vi "DAQ Performance Test.vi"() -> ()   [LabVIEW 2021]
uses:
  <vilib>/Platform/TimedLoop/XDataNode/wakeup.ctl
  <vilib>/Platform/TimedLoop/XDataNode/XDNodeRunTimeDep.lvlib
  <vilib>/Platform/TimedLoop/XDataNode/nitl_modes.ctl
  <vilib>/Platform/TimedLoop/XDataNode/timing_clust.ctl
  <vilib>/Platform/TimedLoop/XDataNode/XDataNode.xnode
  CIFChannels/Typedef/Direction.ctl
  CIFChannels/CIFChannels.lvclass
  ChannelCommon/typedef/FIFO Config.ctl
  ChannelCommon/ChannelCommon.lvlib
  CIF_CIPC_Fifo_DAQ.lvclass
  D:/dev/Packages/CIF_Channels_Core/src/CIPC_Channels/CIF_CIPC_Chan/CIF_CIPC_Chn.lvclass
  D:/dev/Packages/CIF_Channels_Core/src/CIFChannels/CIFChannels.lvclass
  D:/dev/Packages/CIF_Channels_Core/src/CIPC_Channels/FIFO_DAQ/CIF_CIPC_Fifo_DAQ.lvclass
  ChannelCommon/typedef/TimeStamps.ctl
  ChannelCommon/typedef/Datatype Waveform.ctl
  ChannelCommon/typedef/New FIFO Instance Configuration.ctl
  ChannelCommon/typedef/Benchmark Stats.ctl
panel:
  in  "stop":bool
  out "Flatten (us) TO":T1
  out "Channel R/W (us) TO":T1
  out "Flatten (us)":T1
  out "Channel R/W (us)":T1
  out "avg TO":dbl
  out "max TO":dbl
  out "timed out? 3":bool
  out "timed out?":bool
  out "avg channel":dbl
  out "max channel":dbl
  out "pass":bool
  out "error out":errorcluster
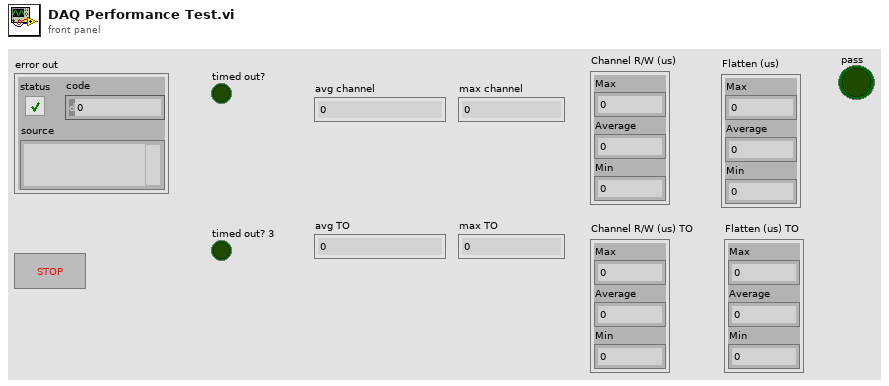
[diagram p1: front panel]
types:
  T1 = typedef "ChannelCommon.lvlib/Benchmark Stats.ctl" = cluster{"Max":i64, "Average":dbl, "Min":i64}
  T2 = typedef "ChannelCommon.lvlib/FIFO Config.ctl" = cluster{"Max Bytes/Msg":u64, "Max Msg/FIFO":u64, "Flags":u64}
  T3 = typedef "CIFChannels.lvclass/Direction.ctl" = enum16{"Publisher", "Subscriber"}
  T4 = typedef "ChannelCommon.lvlib/New FIFO Instance Configuration.ctl" = cluster{"Backpressure":bool, "Bytes/Message Override":u32, "Messages/FIFO Override":u32, "Custom Data":u8[]}
  T5 = typedef "ChannelCommon.lvlib/Datatype Waveform.ctl" = cluster{"Measurement":dbl[], "dT":dbl, "Timestamp":i64}
  T6 = typedef "ChannelCommon.lvlib/TimeStamps.ctl" = cluster{"ClockID":u8, "T0":i64, "T_Out":i64}
  T7 = typedef "XDNodeRunTimeDep.lvlib/timing_clust.ctl" = cluster{"Expected End [f-1]":u64, "Actual End [f-1]":u64, "Finished Late? [f-1]":bool, "Expected End [i-1]":u64, "Actual End [i-1]":u64, "Finished Late? [i-1]":bool, "Expected Start [i]":u64, "Actual Start [i]":u64, "Expected Start [f]":u64, "Actual Start [f]":u64, "Source Name":string, "Structure Name":string, "Period":i64, "Deadline":i64, "Offset":i64, "Start":i64, "Priority":i32, "Timeout":i32, "Mode":T8, "Wakeup Reason":T9, "Error":errorcluster, "Source Type":string, "Secondary Source Type":string, "Global End Time":u64, "Global Start Time":u64, "Frame Duration":u64, "Iteration Duration":u64, "Assigned CPU":i32, "I/O Scan Engine Mode":u32}
  T8 = typedef "XDNodeRunTimeDep.lvlib/nitl_modes.ctl" = enum32{"No Change", "Process missed periods, maintain original phase", "Discard missed periods, maintain original phase", "Process missed periods, ignore original phase", "Discard missed periods, ignore original phase"}
  T9 = typedef "XDNodeRunTimeDep.lvlib/wakeup.ctl" = enum32{"Normal", "Aborted", "Asynchronous wakeup", "Timing source error", "Timed loop error", "Timeout"}
  T10 = typedef "ChannelCommon.lvlib/New FIFO Instance Response.ctl" = cluster{"Publisher":string, "Custom Data":u8[]}
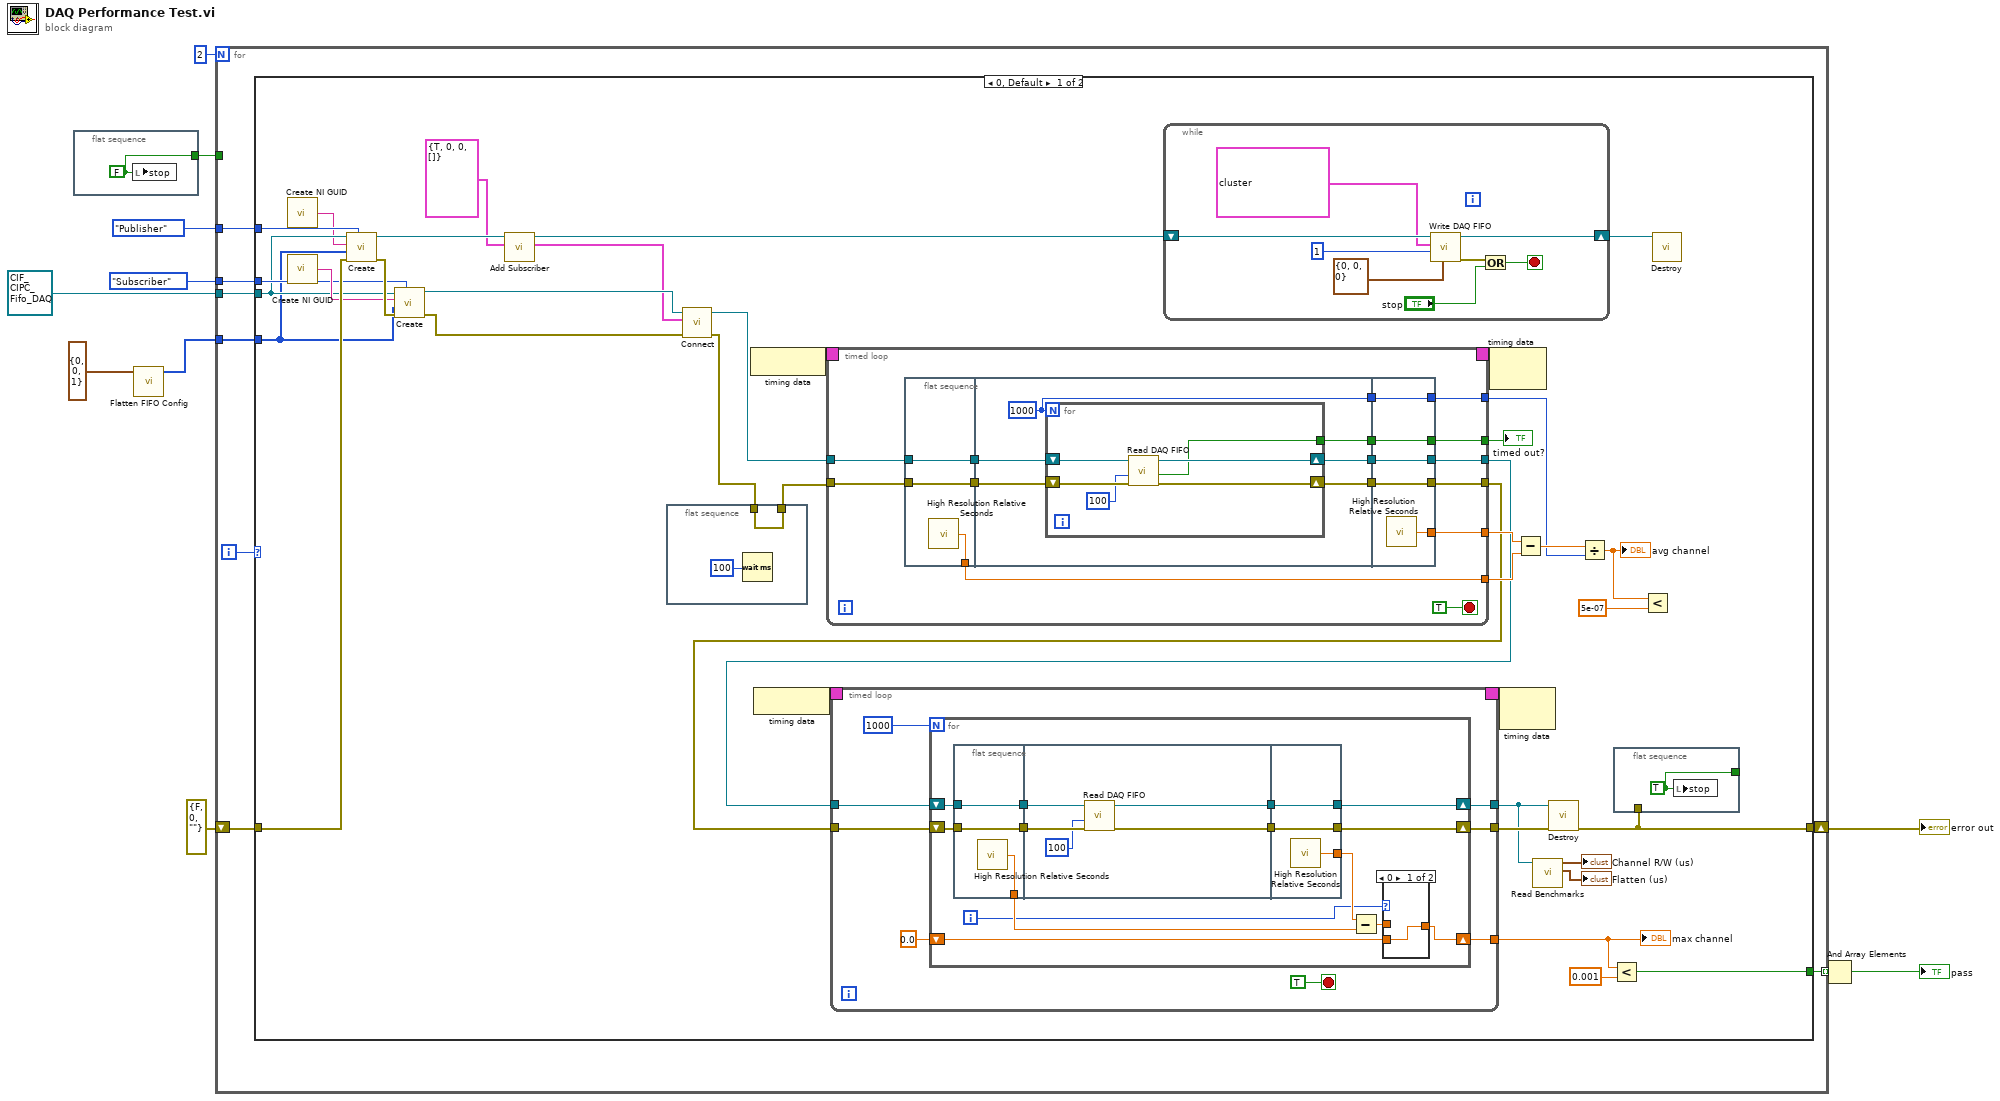
[diagram p0: block diagram]
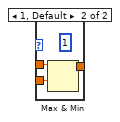
[diagram p2: hidden frame]
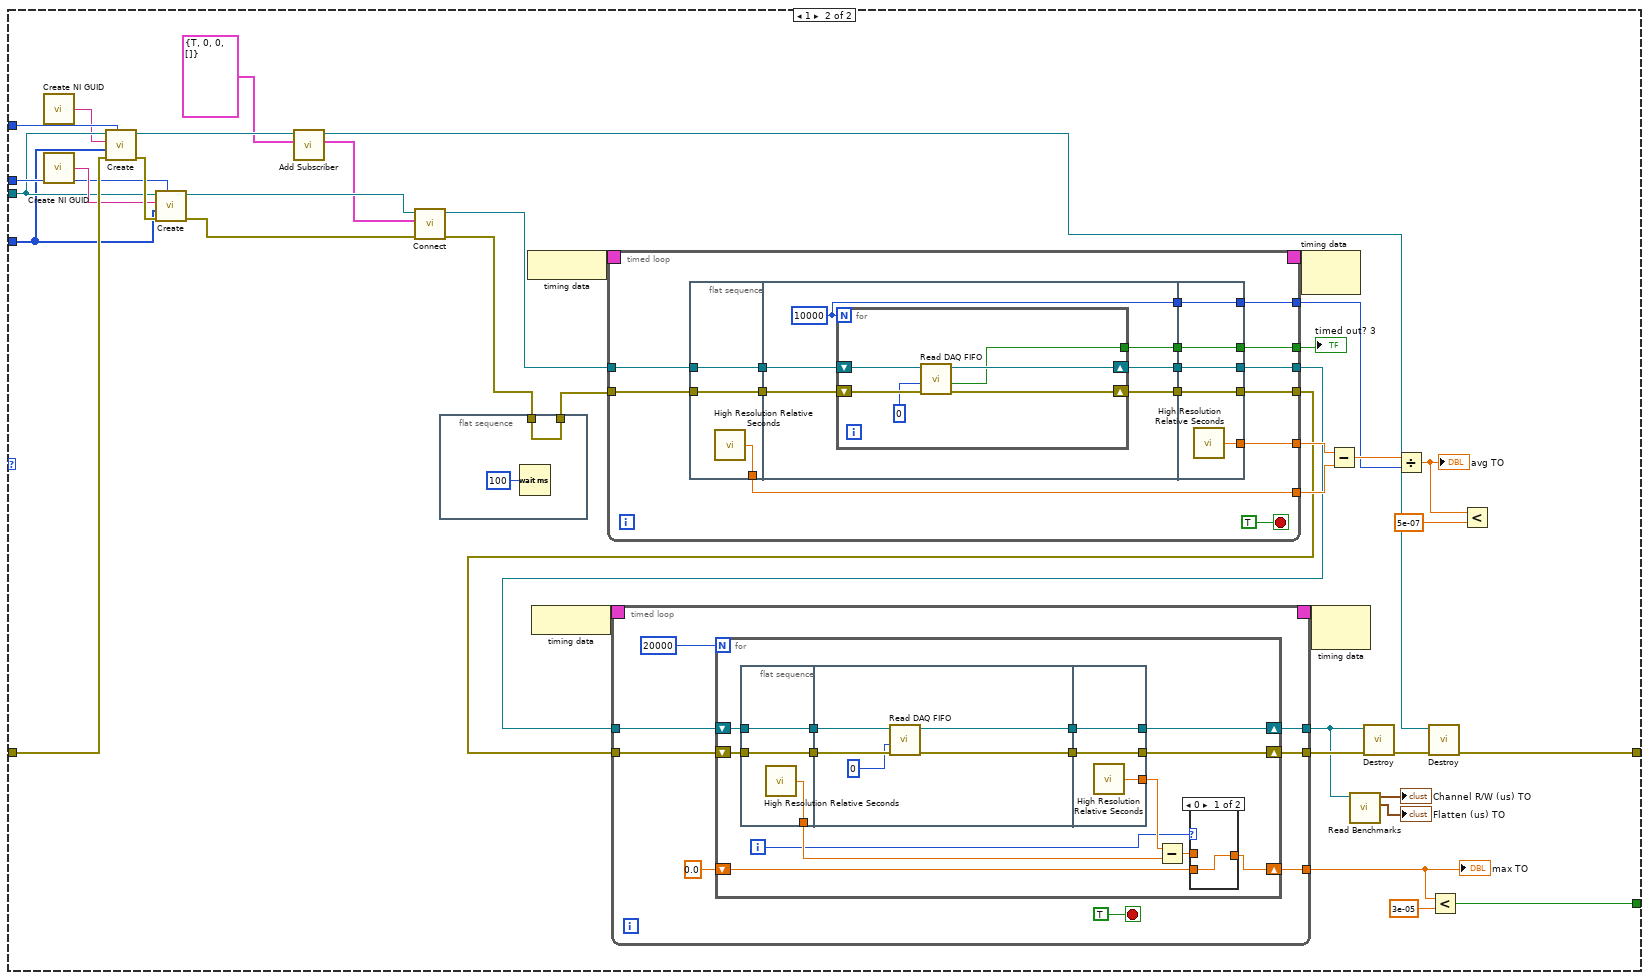
[diagram p3: hidden frame]
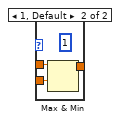
[diagram p4: hidden frame]
diagram:
  n1 = flat-sequence {
    tunnel: [w12] -> w1
    frame #0 {
      w12 = FALSE ("stop")
      n2 = local write "stop"(w12) -> ()
    }
  }
  n3 = call "Flatten FIFO Config.vi"("FIFO Config in"=T2 {"Max Bytes/Msg"=0, "Max Msg/FIFO"=0, "Flags"=1}) -> ("Flattened FIFO Config"=w3:u8[])  [unwired: 10 in]
  n4 = for {
    N: 2 -> [_]
    tunnel: [w20] -> w9 mode=indexing
    shift-right: [w19] -> w11
    shift-left: errorcluster {"status"=FALSE, "code"=0, "source"=""} ("error out") -> [w17]
    tunnel: Direction."Publisher" ("Direction") -> [w16]
    tunnel: Direction."Subscriber" ("Direction") -> [w15]
    tunnel: refnum<class "CIF_CIPC_Fifo_DAQ.lvclass"> refnum ("CIF_CIPC_Fifo_U8.lvclass") -> [w14]
    tunnel: w3 -> [w13]
    tunnel: w1 -> [_]
    i -> [w18]
    n5 = case shown="0, Default" w18 {
      tunnel: [w45 w175] -> w20
      tunnel: [w26 w161] -> w19
      tunnel: w17 -> [w43 w173]
      tunnel: w16 -> [w41 w171]
      tunnel: w15 -> [w40 w170]
      tunnel: w14 -> [w39 w169]
      tunnel: w13 -> [w36 w165]
      frame 0, Default {
        n6 = call <vilib>:"Create NI GUID.vi"() -> ("NI GUID"=w23:string)
        n7 = call <vilib>:"Create NI GUID.vi"() -> ("NI GUID"=w42:string)
        n8 = call-dynamic "Create.vi"("Direction"=w41, "error in (no error)"=w43, "Custom Config Data"=w36, "Name"=w23, "CIFFIFO in"=w39) -> ("error out"=w44:errorcluster, "CIFFIFO out"=w25:refnum<class "CIF_CIPC_Fifo_DAQ.lvclass">)  [unwired: 5 in]
        n9 = call-dynamic "Create.vi"("Direction"=w40, "error in (no error)"=w44, "Custom Config Data"=w36, "Name"=w42, "CIFFIFO in"=w39) -> ("error out"=w37:errorcluster, "CIFFIFO out"=w38:refnum<class "CIF_CIPC_Fifo_DAQ.lvclass">)  [unwired: 5 in]
        n10 = call-dynamic "Add Subscriber.vi"("New FIFO Instance Config"=T4 {"Backpressure"=TRUE, "Bytes/Message Override"=0, "Messages/FIFO Override"=0, "Custom Data"=[]}, "CIF_CIPC_Chn in"=w25) -> ("New FIFO Instance"=w22:T10, "CIF_CIPC_Chn out"=w24:refnum<class "CIF_CIPC_Fifo_DAQ.lvclass">)  [unwired: 7 in, 1 out]
        n11 = flat-sequence {
          tunnel: w33 -> [w62]
          tunnel: [w62] -> w32
          frame #0 {
            n12 = Wait (ms)(milliseconds to wait=u32 100) -> ()  [unwired: 1 out]
          }
        }
        n13 = call-dynamic "Connect.vi"("error in (no error)"=w37, "Connection"=w22, "CIFTag in"=w38) -> ("error out"=w33:errorcluster, "CIFTag out"=w35:refnum<class "CIF_CIPC_Fifo_DAQ.lvclass">)  [unwired: 7 in]
        n14 = node-c288() -> (w59:T7)
        n15 = node-c288() -> (w57:T7)
        n16 = timed-loop {
          timing: w59 -> [_]
          timing-out: [_] -> w58
          tunnel: w35 -> [w126]
          tunnel: w32 -> [w125]
          tunnel: [w121] -> w51
          tunnel: [w119] -> w50
          tunnel: [w117] -> w55
          tunnel: [w116] -> w54
          tunnel: [w115] -> w52
          tunnel: [w113] -> w31
          stop <- TRUE stop-if-true
          n17 = flat-sequence {
            tunnel: w125 -> [w128]
            tunnel: w126 -> [w129]
            tunnel: [w129] -> w123
            tunnel: [w128] -> w122
            tunnel: [w127] -> w116
            tunnel: w123 -> [w135]
            tunnel: w122 -> [w134]
            tunnel: [w133] -> w120
            tunnel: [w132] -> w118
            tunnel: [w131] -> w114
            tunnel: [w130] -> w112
            tunnel: [w146] -> w121
            tunnel: w120 -> [w146]
            tunnel: [w145] -> w119
            tunnel: w118 -> [w145]
            tunnel: [w144] -> w117
            tunnel: [w143] -> w115
            tunnel: w114 -> [w143]
            tunnel: [w142] -> w113
            tunnel: w112 -> [w142]
            frame #0 {
              n18 = call <vilib>:"High Resolution Relative Seconds.vi"() -> ("relative seconds"=w127:dbl)
            }
            frame #1 {
              w131 = 1000
              n19 = for {
                N: w131 -> [_]
                shift-right: [w138] -> w133
                shift-left: w135 -> [w141]
                shift-right: [w139] -> w132
                shift-left: w134 -> [w140]
                tunnel: [w136] -> w130
                n20 = call-dynamic "Read DAQ FIFO.vi"("error in (no error)"=w140, "Timeout (ms)"=100, "CIFFIFO in"=w141) -> ("error out"=w139:errorcluster, "timed out?"=w136:bool, "CIFFIFO out"=w138:refnum<class "CIF_CIPC_Fifo_DAQ.lvclass">)  [unwired: 4 in, 2 out]
              }
            }
            frame #2 {
              n21 = call <vilib>:"High Resolution Relative Seconds.vi"() -> ("relative seconds"=w144:dbl)
            }
          }
        }
        "timed out?" <- w31
        n22 = timed-loop {
          timing: w57 -> [_]
          timing-out: [_] -> w56
          tunnel: w51 -> [w78]
          tunnel: w50 -> [w77]
          tunnel: [w75] -> w30
          tunnel: [w74] -> w34
          tunnel: [w71] -> w47
          stop <- TRUE stop-if-true
          n23 = for {
            N: 1000 -> [_]
            shift-right: [w87] -> w75
            shift-left: w78 -> [w89]
            shift-right: [w86] -> w74
            shift-left: w77 -> [w88]
            shift-right: [w81] -> w71
            shift-left: 0.0 -> [w82]
            i -> [w80]
            n24 = flat-sequence {
              tunnel: w88 -> [w98]
              tunnel: w89 -> [w99]
              tunnel: [w99] -> w92
              tunnel: [w98] -> w91
              tunnel: [w97] -> w84
              tunnel: w92 -> [w104]
              tunnel: w91 -> [w103]
              tunnel: [w101] -> w90
              tunnel: [w102] -> w79
              tunnel: [w107] -> w87
              tunnel: w90 -> [w107]
              tunnel: [w106] -> w86
              tunnel: [w105] -> w85
              tunnel: w79 -> [w106]
              frame #0 {
                n25 = call <vilib>:"High Resolution Relative Seconds.vi"() -> ("relative seconds"=w97:dbl)
              }
              frame #1 {
                n26 = call-dynamic "Read DAQ FIFO.vi"("error in (no error)"=w103, "Timeout (ms)"=100, "CIFFIFO in"=w104) -> ("error out"=w102:errorcluster, "CIFFIFO out"=w101:refnum<class "CIF_CIPC_Fifo_DAQ.lvclass">)  [unwired: 4 in, 3 out]
              }
              frame #2 {
                n27 = call <vilib>:"High Resolution Relative Seconds.vi"() -> ("relative seconds"=w105:dbl)
              }
            }
            n28 = Subtract(x=w85, y=w84) -> (x-y=w83:dbl)
            n29 = case shown="0" w80 {
              tunnel: w83 -> [_ w96]
              tunnel: w82 -> [w93 w95]
              tunnel: [w93 w94] -> w81
              frame 0 {
              }
              frame 1, Default {
                (unwired) u32 1 ("milliseconds to wait")
                n30 = Max & Min(x=w96, y=w95) -> (max(x,y)=w94:dbl)  [unwired: 1 out]
              }
            }
          }
        }
        "max channel" <- w47
        n31 = while {
          shift-right: [w68] -> w27
          shift-left: w24 -> [w70]
          stop <- w66 stop-if-true
          n32 = call-dynamic "Write DAQ FIFO.vi"("FIFO Timestamps"=T6 {"ClockID"=0, "T0"=0, "T_Out"=0}, "Timeout (ms)"=1, "Data In"=T5[] [{"Measurement"=array[100000 elements], "dT"=3.0, "Timestamp"=121}], "CIFFIFO in"=w70) -> ("error out"=w67:errorcluster, "CIFFIFO out"=w68:refnum<class "CIF_CIPC_Fifo_DAQ.lvclass">)  [unwired: 4 in, 2 out]
          n33 = Or(x=w67, y="stop") -> (x .or. y?=w66:bool)
        }
        n34 = node-c288(w58) -> ()  [unwired: 1 out]
        n35 = node-c288(w56) -> ()  [unwired: 1 out]
        n36 = Subtract(x=w55, y=w54) -> (x-y=w53:dbl)
        n37 = call "Read Benchmarks.vi"("CIFChannels in"=w30) -> ("Flatten (us)"=→"Flatten (us)":T1, "Channel R/W (us)"=→"Channel R/W (us)":T1)  [unwired: 9 in]
        n38 = call-dynamic "Destroy.vi"("error in (no error)"=w34, "CIFTag in"=w30) -> ("error out"=w26:errorcluster)  [unwired: 8 in, 1 out]
        n39 = Divide(x=w53, y=w52) -> (x/y=w49:dbl)
        "avg channel" <- w49
        n40 = Less?(x=w47, y=0.001) -> (x < y?=w45:bool)
        n41 = flat-sequence {
          tunnel: [w60] -> _
          tunnel: w26 -> [_]
          frame #0 {
            w60 = TRUE ("stop")
            n42 = local write "stop"(w60) -> ()
          }
        }
        n43 = Less?(x=w49, y=5e-07) -> ()  [unwired: 1 out]
        n44 = call-dynamic "Destroy.vi"("CIFTag in"=w27) -> ()  [unwired: 9 in, 2 out]
      }
      frame 1 {
        n45 = call <vilib>:"Create NI GUID.vi"() -> ("NI GUID"=w167:string)
        n46 = call <vilib>:"Create NI GUID.vi"() -> ("NI GUID"=w172:string)
        n47 = call-dynamic "Create.vi"("Direction"=w171, "error in (no error)"=w173, "Custom Config Data"=w165, "Name"=w167, "CIFFIFO in"=w169) -> ("error out"=w174:errorcluster, "CIFFIFO out"=w154:refnum<class "CIF_CIPC_Fifo_DAQ.lvclass">)  [unwired: 5 in]
        n48 = call-dynamic "Create.vi"("Direction"=w170, "error in (no error)"=w174, "Custom Config Data"=w165, "Name"=w172, "CIFFIFO in"=w169) -> ("error out"=w166:errorcluster, "CIFFIFO out"=w168:refnum<class "CIF_CIPC_Fifo_DAQ.lvclass">)  [unwired: 5 in]
        n49 = call-dynamic "Add Subscriber.vi"("New FIFO Instance Config"=T4 {"Backpressure"=TRUE, "Bytes/Message Override"=0, "Messages/FIFO Override"=0, "Custom Data"=[]}, "CIF_CIPC_Chn in"=w154) -> ("New FIFO Instance"=w152:T10, "CIF_CIPC_Chn out"=w153:refnum<class "CIF_CIPC_Fifo_DAQ.lvclass">)  [unwired: 7 in, 1 out]
        n50 = call-dynamic "Connect.vi"("error in (no error)"=w166, "Connection"=w152, "CIFTag in"=w168) -> ("error out"=w160:errorcluster, "CIFTag out"=w164:refnum<class "CIF_CIPC_Fifo_DAQ.lvclass">)  [unwired: 7 in]
        n51 = flat-sequence {
          tunnel: w160 -> [w191]
          tunnel: [w191] -> w159
          frame #0 {
            n52 = Wait (ms)(milliseconds to wait=u32 100) -> ()  [unwired: 1 out]
          }
        }
        n53 = node-c288() -> (w189:T7)
        n54 = node-c288() -> (w187:T7)
        n55 = timed-loop {
          timing: w189 -> [_]
          timing-out: [_] -> w188
          tunnel: w164 -> [w247]
          tunnel: w159 -> [w246]
          tunnel: [w242] -> w181
          tunnel: [w240] -> w180
          tunnel: [w238] -> w185
          tunnel: [w237] -> w184
          tunnel: [w236] -> w182
          tunnel: [w234] -> w158
          stop <- TRUE stop-if-true
          n56 = flat-sequence {
            tunnel: w246 -> [w249]
            tunnel: w247 -> [w250]
            tunnel: [w250] -> w244
            tunnel: [w249] -> w243
            tunnel: [w248] -> w237
            tunnel: w244 -> [w256]
            tunnel: w243 -> [w255]
            tunnel: [w254] -> w241
            tunnel: [w253] -> w239
            tunnel: [w252] -> w235
            tunnel: [w251] -> w233
            tunnel: [w267] -> w242
            tunnel: w241 -> [w267]
            tunnel: [w266] -> w240
            tunnel: w239 -> [w266]
            tunnel: [w265] -> w238
            tunnel: [w264] -> w236
            tunnel: w235 -> [w264]
            tunnel: [w263] -> w234
            tunnel: w233 -> [w263]
            frame #0 {
              n57 = call <vilib>:"High Resolution Relative Seconds.vi"() -> ("relative seconds"=w248:dbl)
            }
            frame #1 {
              w252 = 10000
              n58 = for {
                N: w252 -> [_]
                shift-right: [w259] -> w254
                shift-left: w256 -> [w262]
                shift-right: [w260] -> w253
                shift-left: w255 -> [w261]
                tunnel: [w258] -> w251
                n59 = call-dynamic "Read DAQ FIFO.vi"("error in (no error)"=w261, "Timeout (ms)"=0, "CIFFIFO in"=w262) -> ("error out"=w260:errorcluster, "timed out?"=w258:bool, "CIFFIFO out"=w259:refnum<class "CIF_CIPC_Fifo_DAQ.lvclass">)  [unwired: 4 in, 2 out]
              }
            }
            frame #2 {
              n60 = call <vilib>:"High Resolution Relative Seconds.vi"() -> ("relative seconds"=w265:dbl)
            }
          }
        }
        "timed out? 3" <- w158
        n61 = timed-loop {
          timing: w187 -> [_]
          timing-out: [_] -> w186
          tunnel: w181 -> [w199]
          tunnel: w180 -> [w198]
          tunnel: [w196] -> w155
          tunnel: [w195] -> w163
          tunnel: [w192] -> w177
          stop <- TRUE stop-if-true
          n62 = for {
            N: 20000 -> [_]
            shift-right: [w208] -> w196
            shift-left: w199 -> [w210]
            shift-right: [w207] -> w195
            shift-left: w198 -> [w209]
            shift-right: [w202] -> w192
            shift-left: 0.0 -> [w203]
            i -> [w201]
            n63 = flat-sequence {
              tunnel: w209 -> [w219]
              tunnel: w210 -> [w220]
              tunnel: [w220] -> w213
              tunnel: [w219] -> w212
              tunnel: [w218] -> w205
              tunnel: w213 -> [w225]
              tunnel: w212 -> [w223]
              tunnel: [w224] -> w211
              tunnel: [w222] -> w200
              tunnel: [w228] -> w208
              tunnel: w211 -> [w228]
              tunnel: [w227] -> w207
              tunnel: [w226] -> w206
              tunnel: w200 -> [w227]
              frame #0 {
                n64 = call <vilib>:"High Resolution Relative Seconds.vi"() -> ("relative seconds"=w218:dbl)
              }
              frame #1 {
                n65 = call-dynamic "Read DAQ FIFO.vi"("error in (no error)"=w223, "Timeout (ms)"=0, "CIFFIFO in"=w225) -> ("error out"=w222:errorcluster, "CIFFIFO out"=w224:refnum<class "CIF_CIPC_Fifo_DAQ.lvclass">)  [unwired: 4 in, 3 out]
              }
              frame #2 {
                n66 = call <vilib>:"High Resolution Relative Seconds.vi"() -> ("relative seconds"=w226:dbl)
              }
            }
            n67 = Subtract(x=w206, y=w205) -> (x-y=w204:dbl)
            n68 = case shown="0" w201 {
              tunnel: w204 -> [_ w217]
              tunnel: w203 -> [w214 w216]
              tunnel: [w214 w215] -> w202
              frame 0 {
              }
              frame 1, Default {
                (unwired) u32 1 ("milliseconds to wait")
                n69 = Max & Min(x=w217, y=w216) -> (max(x,y)=w215:dbl)  [unwired: 1 out]
              }
            }
          }
        }
        "max TO" <- w177
        n70 = node-c288(w188) -> ()  [unwired: 1 out]
        n71 = node-c288(w186) -> ()  [unwired: 1 out]
        n72 = Subtract(x=w185, y=w184) -> (x-y=w183:dbl)
        n73 = call "Read Benchmarks.vi"("CIFChannels in"=w155) -> ("Flatten (us)"=→"Flatten (us) TO":T1, "Channel R/W (us)"=→"Channel R/W (us) TO":T1)  [unwired: 9 in]
        n74 = call-dynamic "Destroy.vi"("error in (no error)"=w163, "CIFTag in"=w155) -> ("error out"=w162:errorcluster)  [unwired: 8 in, 1 out]
        n75 = Divide(x=w183, y=w182) -> (x/y=w179:dbl)
        "avg TO" <- w179
        n76 = call-dynamic "Destroy.vi"("error in (no error)"=w162, "CIFTag in"=w153) -> ("error out"=w161:errorcluster)  [unwired: 8 in, 1 out]
        n77 = Less?(x=w177, y=3e-05) -> (x < y?=w175:bool)
        n78 = Less?(x=w179, y=5e-07) -> ()  [unwired: 1 out]
      }
    }
  }
  "error out" <- w11
  n79 = And Array Elements(Boolean array=w9) -> (logical AND=→"pass":bool)
